vi "test_callback.vi"() -> ()   [LabVIEW 2019]
panel:
  in  "정지":bool
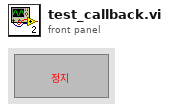
[diagram p1: front panel]
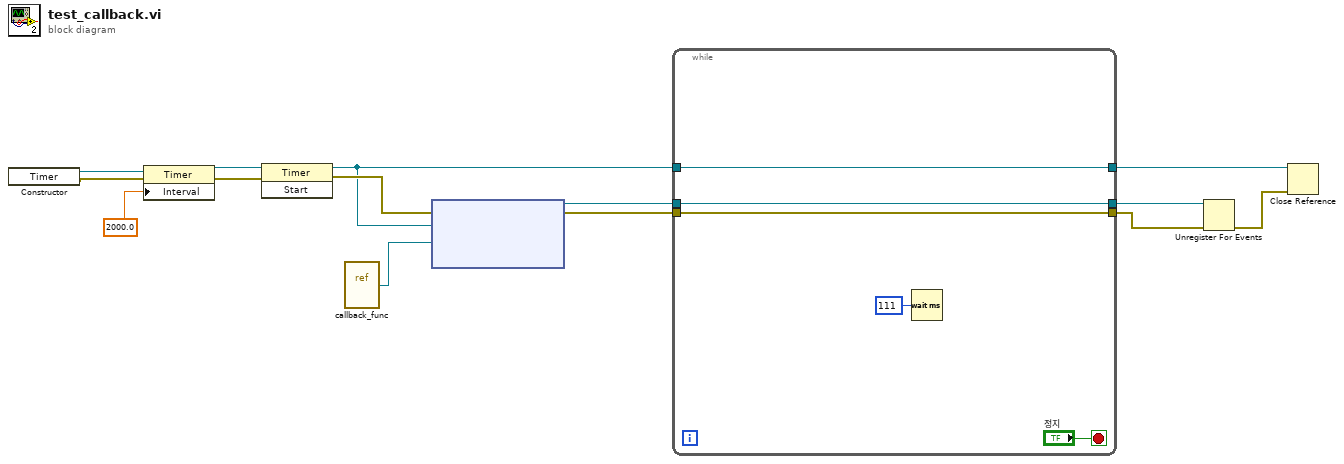
[diagram p0: block diagram]
diagram:
  n1 = constructor class="Timer"() -> (reference out=w14:refnum<k24>, error out=w11:errorcluster)  [unwired: 3 in, 1 out]
  n2 = property on="프로퍼티 노드" class="Timer"(reference=w14, error in=w11, "Interval"=2000.0) -> (reference out=w12:refnum<k24>, error out=w10:errorcluster)
  n3 = invoke on="인보크 노드" class="Timer" method="Start"(reference=w12, error in=w10) -> (reference out=w3:refnum<k24>, error out=w9:errorcluster)  [unwired: 1 in, 1 out]
  n4 = vi-ref "callback_func.vi"() -> ("vi reference"=w8:refnum<vi>)
  n5 = node(w9, w3, w8) -> (w7:refnum<k27>, w6:errorcluster)  [unwired: 2 in]
  n6 = while {
    tunnel: w7 -> [w17]
    tunnel: [w17] -> w5
    tunnel: [w16] -> w2
    tunnel: w6 -> [w16]
    tunnel: [w15] -> w4
    tunnel: w3 -> [w15]
    stop <- "정지" stop-if-true
    n7 = Wait (ms)(milliseconds to wait=u32 111 ("대기 시간 (ms)")) -> ()  [unwired: 1 out]
  }
  n8 = Unregister For Events(event registration refnum=w5, error in=w2) -> (error out=w1:errorcluster)
  n9 = Close Reference(reference=w4, error in (no error)=w1) -> ()  [unwired: 1 out]
